vi "Flush TCP-IP Input Buffer.vi"(5 "TCP/IP ID":refnum<k5>) -> (2 "TCP/IP ID Out":refnum<k5>)   [LabVIEW 2015]
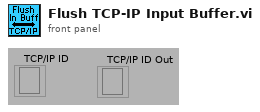
[diagram p1: front panel]
types:
  T1 = enum16{"Standard", "Buffered", "CRLF", "Immediate"}
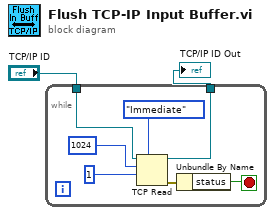
[diagram p0: block diagram]
diagram:
  n1 = while {
    tunnel: "TCP/IP ID" -> [w4]
    tunnel: [w3] -> w1
    stop <- w5 stop-if-true
    n2 = TCP Read(connection ID=w4, bytes to read=1024, 7:T1."Immediate" ("mode (standard)"), 9:1 ("timeout ms (25000)")) -> (connection ID out=w3:refnum<k5>, error out=w6:errorcluster)  [unwired: 1 in, 1 out]
    n3 = Unbundle By Name(w6) -> ("status"=w5:bool)
  }
  "TCP/IP ID Out" <- w1
